vi "midiout_main.vi"   [LabVIEW 2020]
uses:
  midi/midi.lvclass
  <vilib>/Platform/TimedLoop/XDataNode/timing_clust.ctl
  <vilib>/Platform/TimedLoop/XDataNode/nitl_modes.ctl
  <vilib>/Platform/TimedLoop/XDataNode/wakeup.ctl
  d07e9453-c060-4ef9-811b-683eda37ad5b.vi
  midi/midichannel.set.vi
  <vilib>/platform/TimedLoop/XDataNode/XDataNode.xnode
  <vilib>/Platform/TimedLoop/XDataNode/XDNodeRunTimeDep.lvlib
types:
  T1 = typedef "XDNodeRunTimeDep.lvlib/timing_clust.ctl" = cluster{"Expected End [f-1]":u64, "Actual End [f-1]":u64, "Finished Late? [f-1]":bool, "Expected End [i-1]":u64, "Actual End [i-1]":u64, "Finished Late? [i-1]":bool, "Expected Start [i]":u64, "Actual Start [i]":u64, "Expected Start [f]":u64, "Actual Start [f]":u64, "Source Name":string, "Structure Name":string, "Period":i64, "Deadline":i64, "Offset":i64, "Start":i64, "Priority":i32, "Timeout":i32, "Mode":T2, "Wakeup Reason":T3, "Error":errorcluster, "Source Type":string, "Secondary Source Type":string, "Global End Time":u64, "Global Start Time":u64, "Frame Duration":u64, "Iteration Duration":u64, "Assigned CPU":i32, "I/O Scan Engine Mode":u32}
  T2 = typedef "XDNodeRunTimeDep.lvlib/nitl_modes.ctl" = enum32{"No Change", "Process missed periods, maintain original phase", "Discard missed periods, maintain original phase", "Process missed periods, ignore original phase", "Discard missed periods, ignore original phase"}
  T3 = typedef "XDNodeRunTimeDep.lvlib/wakeup.ctl" = enum32{"Normal", "Aborted", "Asynchronous wakeup", "Timing source error", "Timed loop error", "Timeout"}
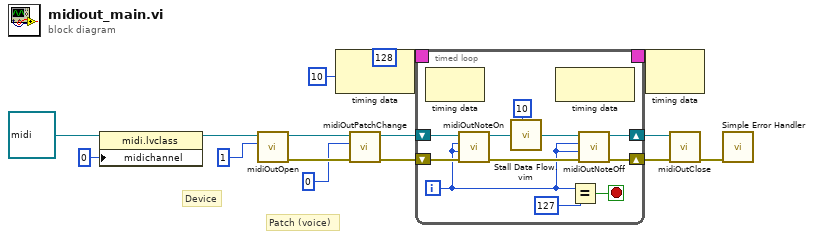
[diagram p0: block diagram]
diagram:
  (unwired) 128
  # "Patch (voice)"
  # "Device"
  n1 = property class="midi.lvclass"(reference=refnum<class "midi.lvclass"> refnum ("midi in"), "midichannel"=u64 0) -> (reference out=w6:refnum<class "midi.lvclass">)  [unwired: 1 in, 1 out]
  n2 = call "midiOutOpen.vi"("DeviceID"=u32 1, "midi in"=w6) -> ("error out"=w8:errorcluster, "midi out"=w11:refnum<class "midi.lvclass">)  [unwired: 8 in]
  n3 = node-c288(i64 10 ("Period")) -> (w3:T1)
  n4 = call "midiOutPatchChange.vi"("error in"=w8, "Patch"=u32 0, "midi in"=w11) -> ("error out"=w9:errorcluster, "midi out"=w10:refnum<class "midi.lvclass">)  [unwired: 7 in]
  n5 = timed-loop {
    shift-right: [w19] -> w12
    shift-left: w10 -> [w24]
    shift-right: [w21] -> w13
    shift-left: w9 -> [w23]
    timing: w3 -> [_]
    timing-out: [_] -> w2
    i -> [w18]
    stop <- w16 stop-if-true
    n6 = node-c288() -> ()  [unwired: 1 in, 1 out]
    n7 = call "midiOutNoteOn.vi"("error in"=w23, "Velocity (0-127)"=w18, "Note (0-127)"=w18, "midi in"=w24) -> ("error out"=w20:errorcluster, "midi out"=w26:refnum<class "midi.lvclass">)  [unwired: 6 in]
    n8 = call "Stall Data Flow.vim"("value in"=w26, "milliseconds to wait"=u32 10) -> ("value out"=w22:refnum<class "midi.lvclass">)  [unwired: 1 out]
    n9 = node-c288() -> ()  [unwired: 1 in, 1 out]
    n10 = Equal?(x=w18, y=127) -> (x = y?=w16:bool)
    n11 = call "midiOutNoteOff.vi"("error in"=w20, "Velocity (0-127)"=w18, "Note (0-127)"=w18, "midi in"=w22) -> ("error out"=w21:errorcluster, "midi out"=w19:refnum<class "midi.lvclass">)  [unwired: 6 in]
  }
  n12 = node-c288(w2) -> ()  [unwired: 1 out]
  n13 = call "midiOutClose.vi"("error in"=w13, "midi in"=w12) -> ("error out"=w15:errorcluster)  [unwired: 8 in, 1 out]
  n14 = call <vilib>:"Simple Error Handler.vi"("error in (no error)"=w15) -> ()  [unwired: 4 in, 5 out]
